vi "Test Suite List Contains only Active Methods.vi"(8 "error in (no error)":errorcluster, 11 "Test Case In":refnum<class "LUnit Test Suite Tests.lvclass">) -> (0 "error out":errorcluster, 3 "Test Case Out":refnum<class "LUnit Test Suite Tests.lvclass">)   [LabVIEW 2020, in "LUnit Test Suite Tests.lvclass"]
uses:
  LUnit Test Suite Tests.lvclass
  C:/Program Files (x86)/National Instruments/LabVIEW 2020/vi.lib/Astemes/LUnit/Test Case.lvclass
  Test Doubles/Test Case Test Double Child/Light Test Case Double.lvclass
  C:/git/astemes-lunit/source/API/LUnit Test Case/LUnit Test Case.lvclass
  <vilib>/Astemes/LUnit/Test Case.lvclass/Test Case.ctl
  59ab914e-4c24-4f3b-92f7-fd9a0f9d0912.vi
  <vilib>/Astemes/LUnit/Append Pass Result.vi
  <vilib>/Astemes/LUnit/Append Fail Result.vi
  <vilib>/Astemes/LUnit/Compare Variants.vi
  <vilib>/Astemes/LUnit/Describe Comparison.vi
  <vilib>/Astemes/LUnit/Variant to string.vi
  <vilib>/Utility/Data Type/Get Type Information.vi
  <vilib>/Utility/LVClass/Get LV Class Name.vi
  source/API/LUnit Test Suite/LUnit Test Suite.lvclass
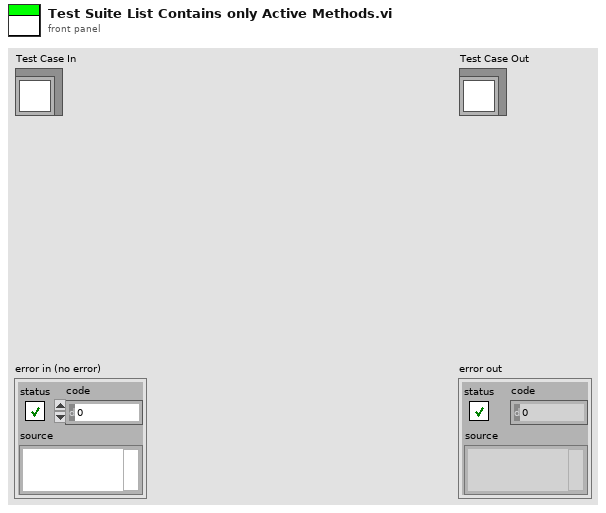
[diagram p1: front panel]
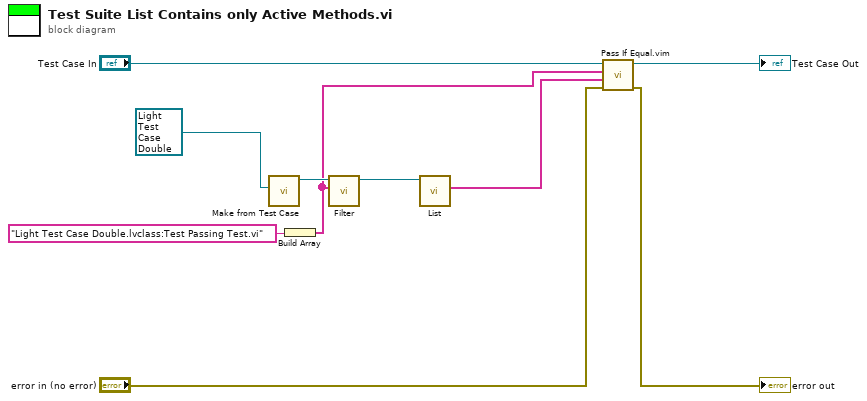
[diagram p0: block diagram]
diagram:
  n1 = call "Make from Test Case.vi"("LUnit Test Case"=refnum<class "Light Test Case Double.lvclass"> refnum ("Light Test Case Double.lvclass")) -> ("LUnit Test Suite Out"=w6:refnum<class "LUnit Test Suite.lvclass">)  [unwired: 9 in, 1 out]
  n2 = Build Array("Light Test Case Double.lvclass:Test Passing Test.vi" ("Methods")) -> (w1:string[])
  n3 = call-dynamic "Filter.vi"("Selected Runnables"=w1, "LUnit Test Suite In"=w6) -> ("LUnit Test Suite Out"=w4:refnum<class "LUnit Test Suite.lvclass">)  [unwired: 8 in, 1 out]
  n4 = call-dynamic "List.vi"("LUnit Test Suite In"=w4) -> ("List of Runnables"=w2:string[])  [unwired: 9 in, 1 out]
  n5 = call "Pass If Equal.vim"("error in (no error)"="error in (no error)", "Actual"=w2, "Expected"=w1, "LUnit Test Case In"="Test Case In") -> ("error out"=→"error out":errorcluster, "LUnit Test Case Out"=→"Test Case Out":refnum<class "LUnit Test Suite Tests.lvclass">)  [unwired: 6 in]
